vi "泵温度校准配置.vi"() -> ()   [LabVIEW 2016, in "斯坦道CODMn新电路板.lvlib"]
uses:
  <vilib>/Utility/miscctls.llb/LVPointTypeDef.ctl
panel:
  in  "关闭":bool
  in  "偏心轮校准簇":T1={"复位"=FALSE, "进水样"=FALSE, "停止"=FALSE, "液体重量"=60, "偏心轮校准"=FALSE}
  in  "温度校准簇":T2={"进水样"=FALSE, "排液"=FALSE, "停止 2"=FALSE, "开始加热"=FALSE, "温度值"=115.0, "温度校准"=FALSE}
  # "偏心轮、温度校准"
  # "输入实际液体重量:"
  # "g"
  # "温度:"
  # "℃"
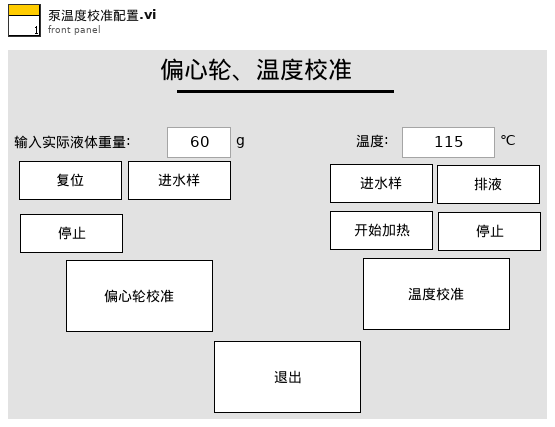
[diagram p1: front panel]
types:
  T1 = cluster{"复位":bool, "进水样":bool, "停止":bool, "液体重量":u16, "偏心轮校准":bool}
  T2 = cluster{"进水样":bool, "排液":bool, "停止 2":bool, "开始加热":bool, "温度值":dbl, "温度校准":bool}
  T3 = typedef "LVPointTypeDef.ctl" = cluster{"Horizontal":i16, "Vertical":i16}
  T4 = cluster{"泵类型":u8, "阀数量":u8, "纯水通道":u8, "废液通道":u8, "进样速度":u16, "出样速度":u16, "滴定速度":u16, "注射泵保温温度L":u8, "注射泵保温温度H":u8, "注射泵加热超时时间":u16, "是否存在液位检测板":u16, "A值告警下限值":u16, "A值告警上限值":u16, "B值告警下限值":u16, "B值告警上限值":u16, "AB跨度告警值":u16, "阀配置:":u8}
  T5 = cluster{"系统时间":timestamp, "工作状态":u16, "测量模式":enum16{"待机", "连续模式", "周期模式", "定点模式", "受控模式", "手动模式"}, "告警代码":u16, "故障代码":u16, "日志代码":u16, "软件版本":u16, "A":sgl, "B":sgl, "K":sgl, "当前滴定数":sgl, "T":sgl, "H":sgl, "id":u16, "flowid":u16, "量程":u16, "加热实时温度":sgl, "当前ORP值":sgl, "运行时间":sgl, "当前步骤剩余时间":sgl, "结束滴定数":sgl, "注射泵保温温度":sgl}
  T6 = cluster{"偏心轮校准参数":dbl, "运行速度(修改需要重启)":u16, "加热温度(校准参数) ":dbl, "告警温度":dbl, "加热超时时间:(单位/秒)":dbl, "K p":dbl, "K i":dbl, "K d":dbl, "ILimitUp":dbl, "ILimitDown":dbl}
  T7 = cluster{"检出限":dbl, "测量精度":dbl, "上限":dbl, "下限":dbl, "阈值（低->高）":dbl, "阈值（高->低）":dbl}
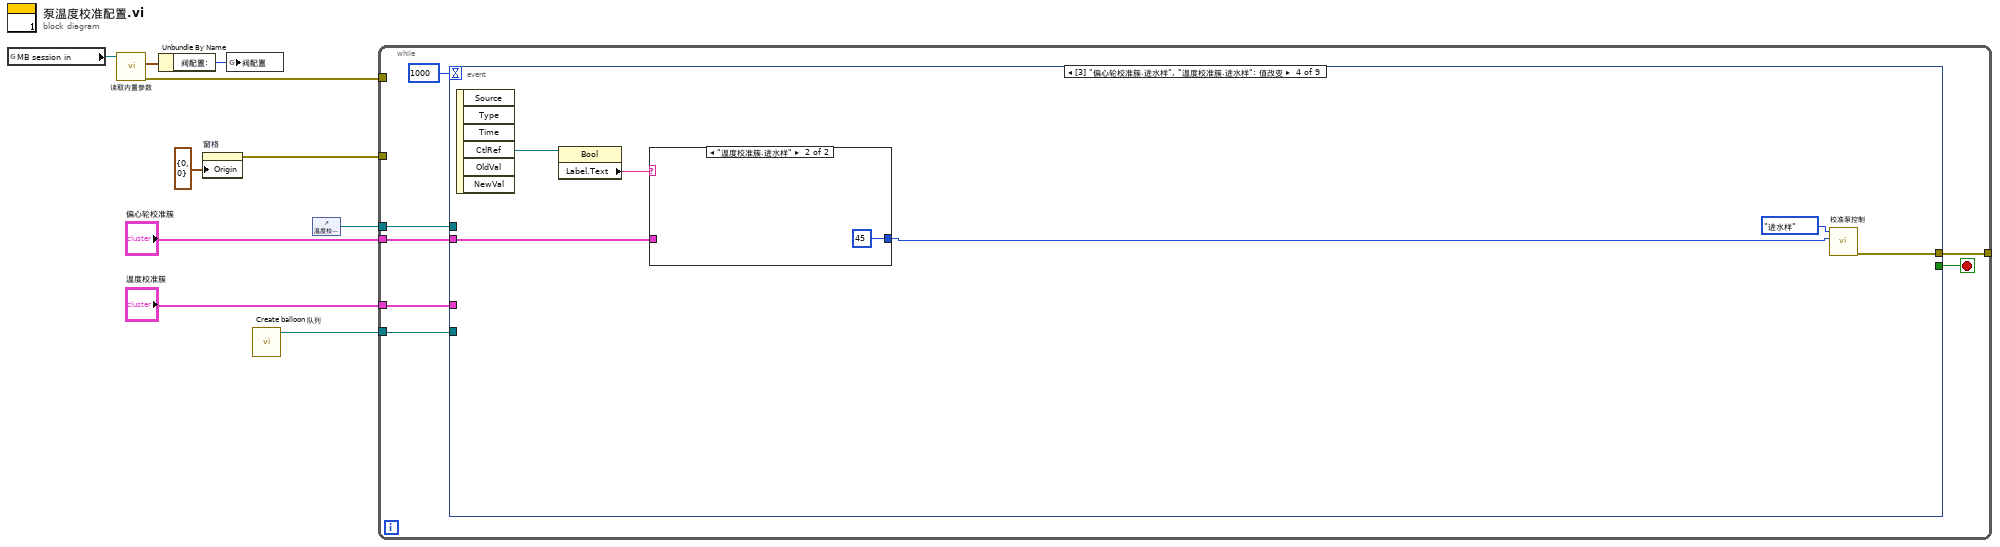
[diagram p0: block diagram]
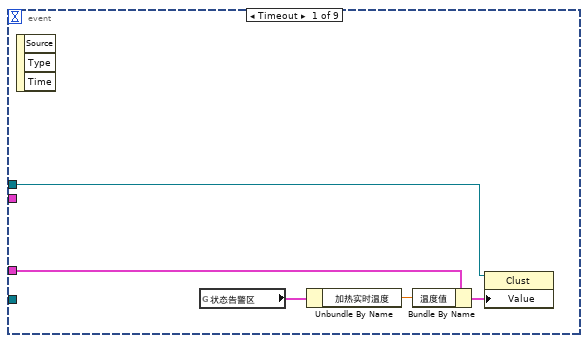
[diagram p2: hidden frame]
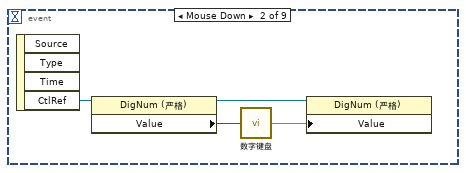
[diagram p3: hidden frame]
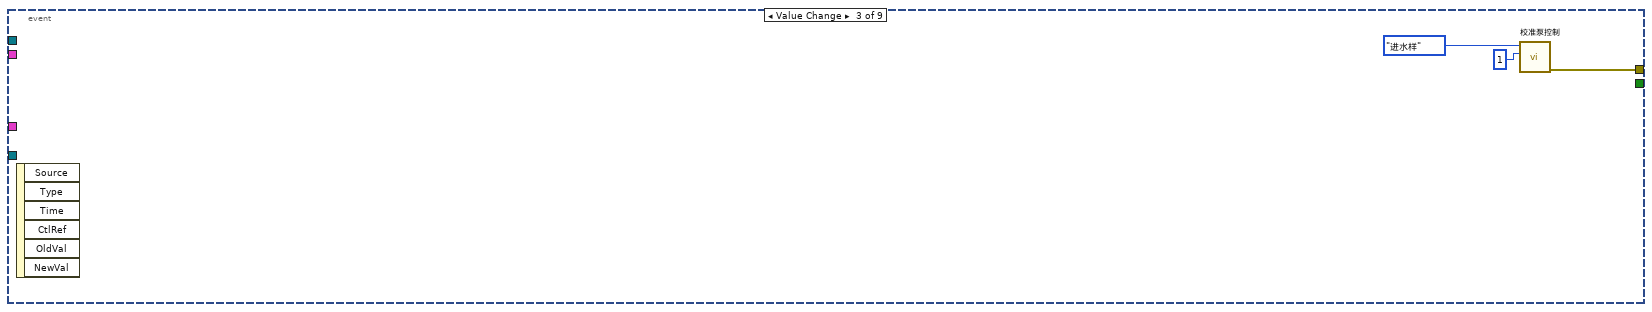
[diagram p4: hidden frame]
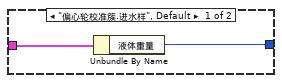
[diagram p5: hidden frame]
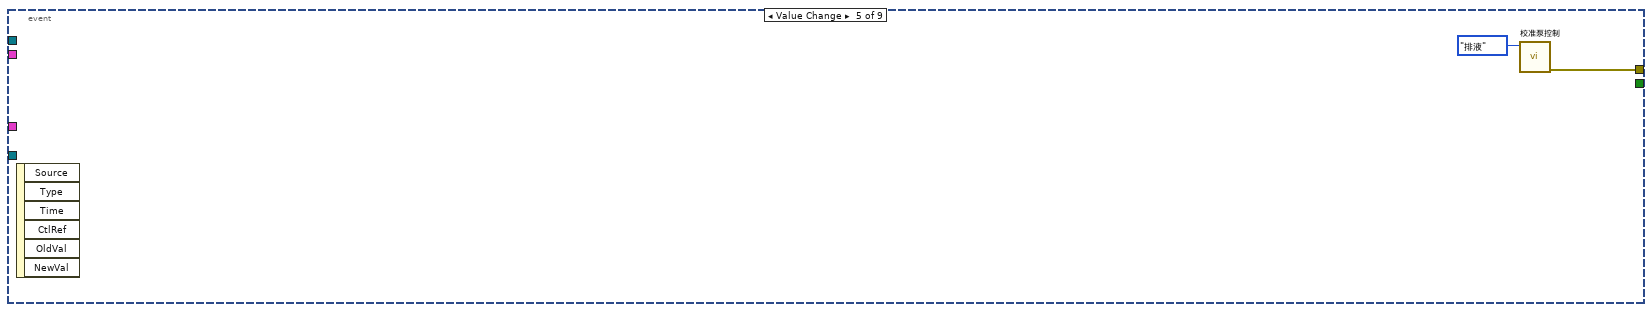
[diagram p6: hidden frame]
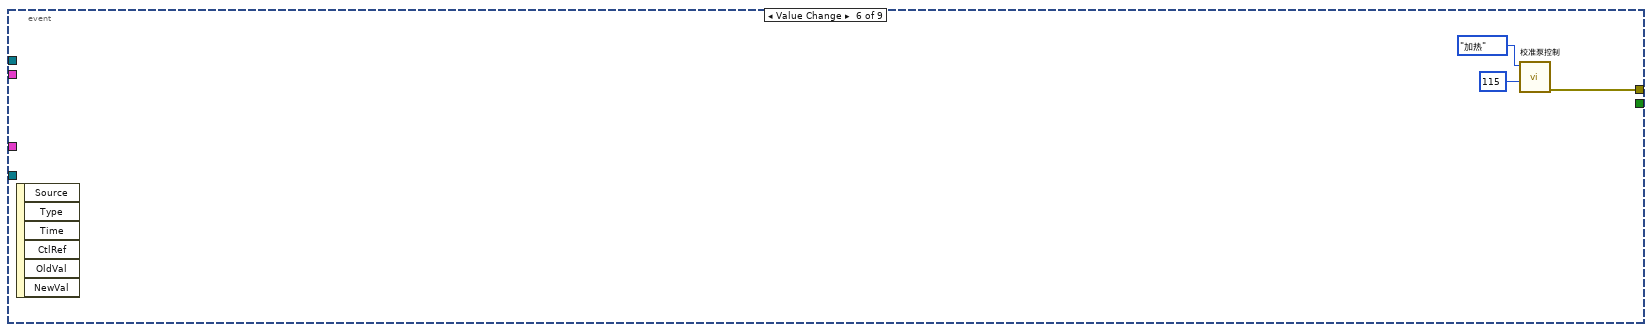
[diagram p7: hidden frame]
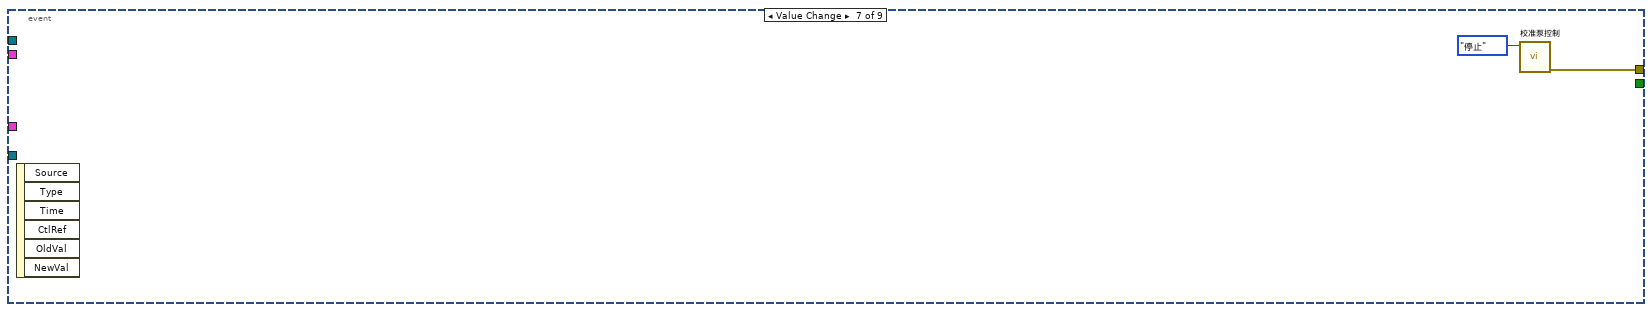
[diagram p8: hidden frame]
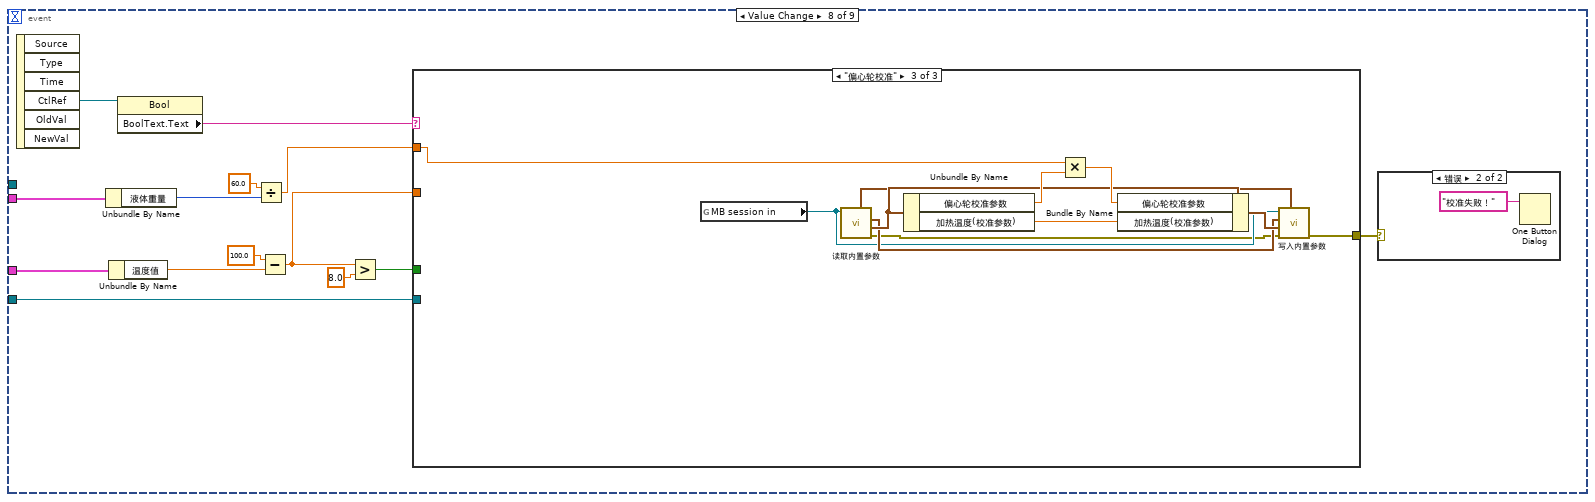
[diagram p9: hidden frame]
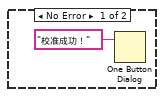
[diagram p10: hidden frame]
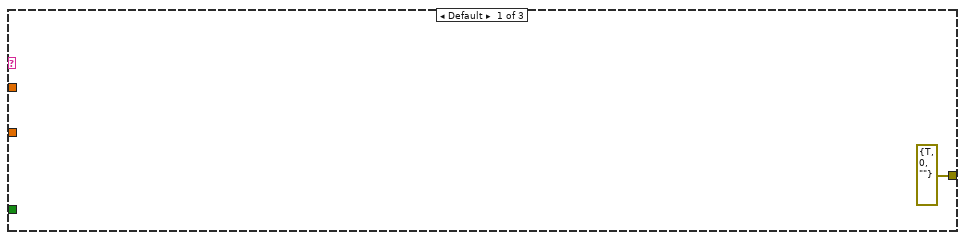
[diagram p11: hidden frame]
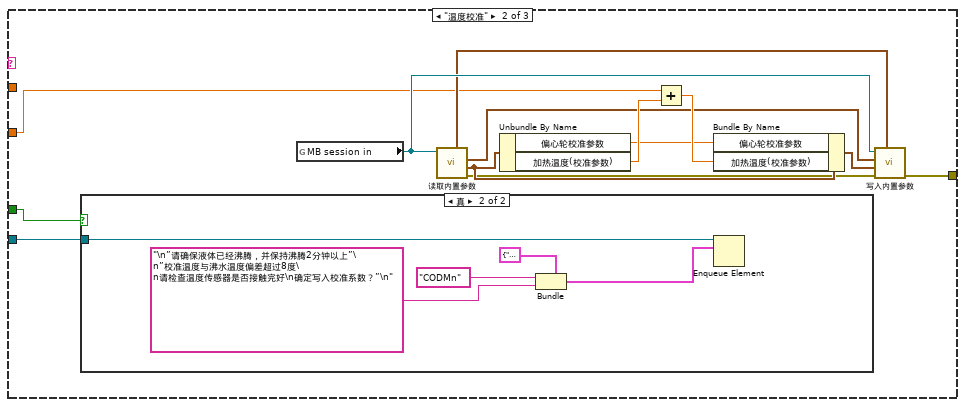
[diagram p12: hidden frame]
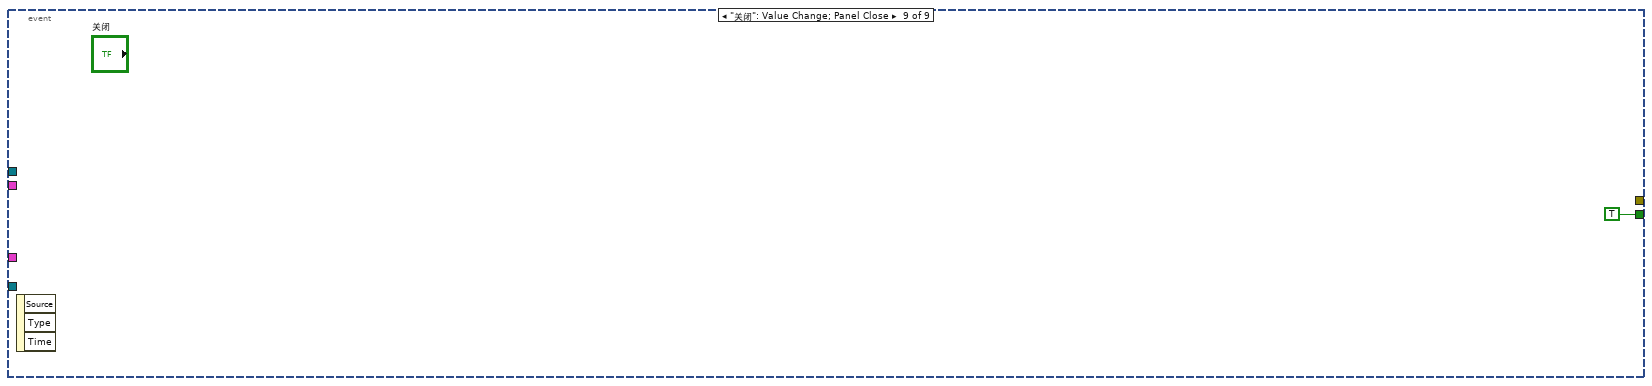
[diagram p14: hidden frame]
diagram:
  n1 = global read "VARCODMn全局变量.vi" "MB session in"() -> (w4:refnum<class "MB_Master.lvclass">)
  n2 = call "读取内置参数.vi"("MB session in"=w4) -> ("error out"=w1:errorcluster, "外设配置"=w3:T4)  [unwired: 6 in, 3 out]
  n3 = Unbundle By Name(w3) -> ("阀配置:"=w2:u8)
  n4 = property on="窗格" class="Pane"("Origin"=T3 {"Horizontal"=0, "Vertical"=0} ("原点")) -> (error out=w10:errorcluster)  [unwired: 2 in, 1 out]
  n5 = global write "CODMn断电保存全局变量.vi" "阀配置"(w2) -> ()
  n6 = call "Create balloon 队列.vi"() -> ("队列输出"=w5:refnum<queue>)  [unwired: 11 in]
  n7 = control-ref of="温度校准簇"() -> (w6:refnum<vi>)
  n8 = while {
    tunnel: w10 -> [_]
    tunnel: "偏心轮校准簇" -> [w16]
    tunnel: [w15] -> _
    tunnel: "温度校准簇" -> [w14]
    tunnel: w6 -> [w12]
    tunnel: w5 -> [w11]
    tunnel: w1 -> [_]
    stop <- w17 stop-if-true
    n9 = event shown="[3] \"偏心轮校准簇.进水样\", \"温度校准簇.进水样\": 值改变" {
      selector: _ -> [_ _ _ _ _ _ _ _ _]
      dyn-events: _ -> [_ _ _ _ _ _ _ _ _]
      timeout: 1000 -> [_ _ _ _ _ _ _ _ _]
      tunnel: [_ _ _ _ _ _ _ _ TRUE] -> w17
      tunnel: w16 -> [_ _ _ w31 _ _ _ w59 _]
      tunnel: [_ _ w27 w34 w39 w42 w44 _ _] -> w15
      tunnel: w14 -> [w21 _ _ _ _ _ _ w57 _]
      tunnel: w12 -> [w19 _ _ _ _ _ _ _ _]
      tunnel: w11 -> [_ _ _ _ _ _ _ w47 _]
      event Timeout {
        n10 = event-data() -> ()  [unwired: 1 in, 3 out]
        n11 = global read "VARCODMn全局变量.vi" "状态告警区"() -> (w22:T5)
        n12 = Unbundle By Name(w22) -> ("加热实时温度"=w20:sgl)
        n13 = Bundle By Name(cluster=w21, "温度值"=w20) -> (w18:T2)
        n14 = property class="Clust"(reference=w19, "Value"=w18) -> ()  [unwired: 1 in, 2 out]
      }
      event "偏心轮校准簇.液体重量": Mouse Down {
        n15 = event-data() -> ("CtlRef"=w23:refnum<vi>)  [unwired: 1 in, 3 out]
        n16 = property class="DigNum (严格)"(reference=w23) -> (reference out=w25:refnum<vi>, "Value"=w26:u16)  [unwired: 1 in, 1 out]
        n17 = call "数字键盘.vi"("OldNumber"=w26) -> ("NewNumber"=w24:dbl)
        n18 = property class="DigNum (严格)"(reference=w25, "Value"=w24) -> ()  [unwired: 1 in, 2 out]
      }
      event "偏心轮校准簇.复位": Value Change {
        n19 = event-data() -> ()  [unwired: 1 in, 6 out]
        n20 = call "校准泵控制.vi"("偏心轮"=u16 1, "枚举"=enum16{"进水样", "排液", "加热", "停止"}."进水样") -> ("错误输出"=w27:errorcluster)  [unwired: 9 in]
      }
      event "偏心轮校准簇.进水样", "温度校准簇.进水样": Value Change {
        n21 = event-data() -> ("CtlRef"=w33:refnum<vi>)  [unwired: 1 in, 5 out]
        n22 = property class="Bool"(reference=w33) -> ("Label.Text"=w32:string)  [unwired: 1 in, 2 out]
        n23 = case shown="\"温度校准簇.进水样\"" w32 {
          tunnel: w31 -> [w37 _]
          tunnel: [w36 u16 45 ("液体重量")] -> w30
          frame "偏心轮校准簇.进水样", Default {
            n24 = Unbundle By Name(w37) -> ("液体重量"=w36:u16)
          }
          frame "温度校准簇.进水样" {
          }
        }
        n25 = call "校准泵控制.vi"("偏心轮"=w30, "枚举"=enum16{"进水样", "排液", "加热", "停止"}."进水样") -> ("错误输出"=w34:errorcluster)  [unwired: 9 in]
      }
      event "温度校准簇.排液": Value Change {
        n26 = event-data() -> ()  [unwired: 1 in, 6 out]
        n27 = call "校准泵控制.vi"("枚举"=enum16{"进水样", "排液", "加热", "停止"}."排液") -> ("错误输出"=w39:errorcluster)  [unwired: 10 in]
      }
      event "温度校准簇.开始加热": Value Change {
        n28 = event-data() -> ()  [unwired: 1 in, 6 out]
        n29 = call "校准泵控制.vi"("摄氏度"=u16 115, "枚举"=enum16{"进水样", "排液", "加热", "停止"}."加热") -> ("错误输出"=w42:errorcluster)  [unwired: 9 in]
      }
      event "温度校准簇.停止 2", "偏心轮校准簇.停止": Value Change {
        n30 = event-data() -> ()  [unwired: 1 in, 6 out]
        n31 = call "校准泵控制.vi"("枚举"=enum16{"进水样", "排液", "加热", "停止"}."停止") -> ("错误输出"=w44:errorcluster)  [unwired: 10 in]
      }
      event "偏心轮校准簇.偏心轮校准", "温度校准簇.温度校准": Value Change {
        n32 = event-data() -> ("CtlRef"=w52:refnum<vi>)  [unwired: 1 in, 5 out]
        n33 = Unbundle By Name(w59) -> ("液体重量"=w56:u16)
        n34 = Unbundle By Name(w57) -> ("温度值"=w54:dbl)
        n35 = property class="Bool"(reference=w52) -> ("BoolText.Text"=w49:string)  [unwired: 1 in, 2 out]
        n36 = Divide(x=60.0, y=w56) -> (x/y=w51:dbl)
        n37 = Subtract(x=100.0, y=w54) -> (x-y=w50:dbl)
        n38 = Greater?(x=w50, y=8.0) -> (0:w48:bool)
        n39 = case shown="\"偏心轮校准\"" w49 {
          tunnel: w51 -> [_ _ w83]
          tunnel: w50 -> [_ w65 _]
          tunnel: w48 -> [_ w67 _]
          tunnel: w47 -> [_ w66 _]
          tunnel: [errorcluster {"status"=TRUE, "code"=0, "source"=""} ("error out") w63 w81] -> w46
          frame Default {
          }
          frame "温度校准" {
            n40 = case shown="真" w67 {
              tunnel: w66 -> [_ w80]
              frame False {
              }
              frame True {
                n41 = Bundle(cluster=cluster{"Title":string, "Body":string} {"Title"="", "Body"=""} ("元素"), "Title"="CODMn", "Body"="\n”请确保液体已经沸腾，并保持沸腾2分钟以上”\n”校准温度与沸水温度偏差超过8度\n请检查温度传感器是否接触完好\n确定写入校准系数？”\n") -> (w76:cluster{"Title":string, "Body":string})
                n42 = Enqueue Element(queue=w80, element=w76) -> ()  [unwired: 2 in, 3 out]
              }
            }
            n43 = global read "VARCODMn全局变量.vi" "MB session in"() -> (w70:refnum<class "MB_Master.lvclass">)
            n44 = call "读取内置参数.vi"("MB session in"=w70) -> ("error out"=w68:errorcluster, "float"=w72:T6, "外设配置"=w71:T4, "量程参数读取"=w69:T7)  [unwired: 6 in, 1 out]
            n45 = Unbundle By Name(w72) -> ("偏心轮校准参数"=w64:dbl, "加热温度(校准参数)"=w74:dbl)
            n46 = Add(x=w65, y=w74) -> (x+y=w75:dbl)
            n47 = Bundle By Name(cluster=w72, "偏心轮校准参数"=w64, "加热温度(校准参数)"=w75) -> (w73:T6)
            n48 = call "写入内置参数.vi"("量程参数读取"=w69, "error in (no error)"=w68, "float"=w73, "外设配置"=w71, "MB session in"=w70) -> ("error out"=w63:errorcluster)  [unwired: 5 in, 1 out]
          }
          frame "偏心轮校准" {
            n49 = global read "VARCODMn全局变量.vi" "MB session in"() -> (w86:refnum<class "MB_Master.lvclass">)
            n50 = call "读取内置参数.vi"("MB session in"=w86) -> ("error out"=w84:errorcluster, "float"=w88:T6, "外设配置"=w87:T4, "量程参数读取"=w85:T7)  [unwired: 6 in, 1 out]
            n51 = Unbundle By Name(w88) -> ("偏心轮校准参数"=w90:dbl, "加热温度(校准参数)"=w82:dbl)
            n52 = Multiply(x=w83, y=w90) -> (x*y=w91:dbl)
            n53 = Bundle By Name(cluster=w88, "偏心轮校准参数"=w91, "加热温度(校准参数)"=w82) -> (w89:T6)
            n54 = call "写入内置参数.vi"("量程参数读取"=w85, "error in (no error)"=w84, "float"=w89, "外设配置"=w87, "MB session in"=w86) -> ("error out"=w81:errorcluster)  [unwired: 5 in, 1 out]
          }
        }
        n55 = case shown="错误" w46 {
          frame No Error {
            n56 = One Button Dialog(message="校准成功！" ("消息")) -> ()  [unwired: 1 in, 1 out]
          }
          frame Error {
            n57 = One Button Dialog(message="校准失败！" ("消息")) -> ()  [unwired: 1 in, 1 out]
          }
        }
      }
      event "关闭": Value Change; Panel Close {
        n58 = event-data() -> ()  [unwired: 1 in, 3 out]
      }
    }
  }
